vi "XY图（绘制多条XY图曲线）.vi"() -> ()   [LabVIEW 2017]
uses:
  <vilib>/Analysis/NI_AALBase.lvlib
panel:
  in  "停止":bool
  out "XY图":cluster{"sine wave":dbl[], "sine wave":dbl[]}[](graph)
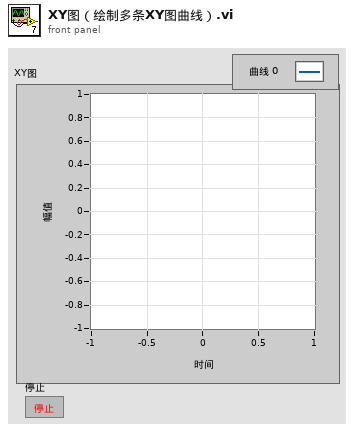
[diagram p1: front panel]
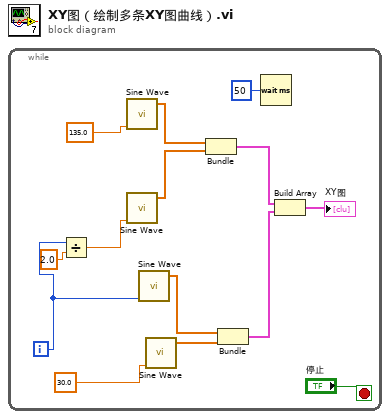
[diagram p0: block diagram]
diagram:
  n1 = while {
    i -> [w13]
    stop <- "停止" stop-if-true
    n2 = Divide(x=w13, y=2.0) -> (x/y=w6:dbl)
    n3 = call <vilib>:"Sine Wave.vi"("phase in"=135.0) -> ("sine wave"=w9:dbl[])  [unwired: 4 in, 2 out]
    n4 = call <vilib>:"Sine Wave.vi"("phase in"=w6) -> ("sine wave"=w8:dbl[])  [unwired: 4 in, 2 out]
    n5 = call <vilib>:"Sine Wave.vi"("phase in"=w13) -> ("sine wave"=w11:dbl[])  [unwired: 4 in, 2 out]
    n6 = call <vilib>:"Sine Wave.vi"("phase in"=30.0) -> ("sine wave"=w10:dbl[])  [unwired: 4 in, 2 out]
    n7 = Bundle("sine wave"=w9, "sine wave"=w8) -> (w4:cluster{"sine wave":dbl[], "sine wave":dbl[]})  [unwired: 1 in]
    n8 = Bundle("sine wave"=w11, "sine wave"=w10) -> (w3:cluster{"sine wave":dbl[], "sine wave":dbl[]})  [unwired: 1 in]
    n9 = Wait (ms)(milliseconds to wait=u32 50 ("等待时间（毫秒）")) -> ()  [unwired: 1 out]
    n10 = Build Array(w4, w3) -> (→"XY图":cluster{"sine wave":dbl[], "sine wave":dbl[]}[])
  }
